vi "prep_outgoing_lineitem.vi"(2 "response":T1, 5 "error in (no error)":errorcluster) -> (15 "to_java":string, 17 "to_terminal":string, 19 "error out":errorcluster)   [LabVIEW 2016]
uses:
  controls/response.ctl
  controls/response_type.ctl
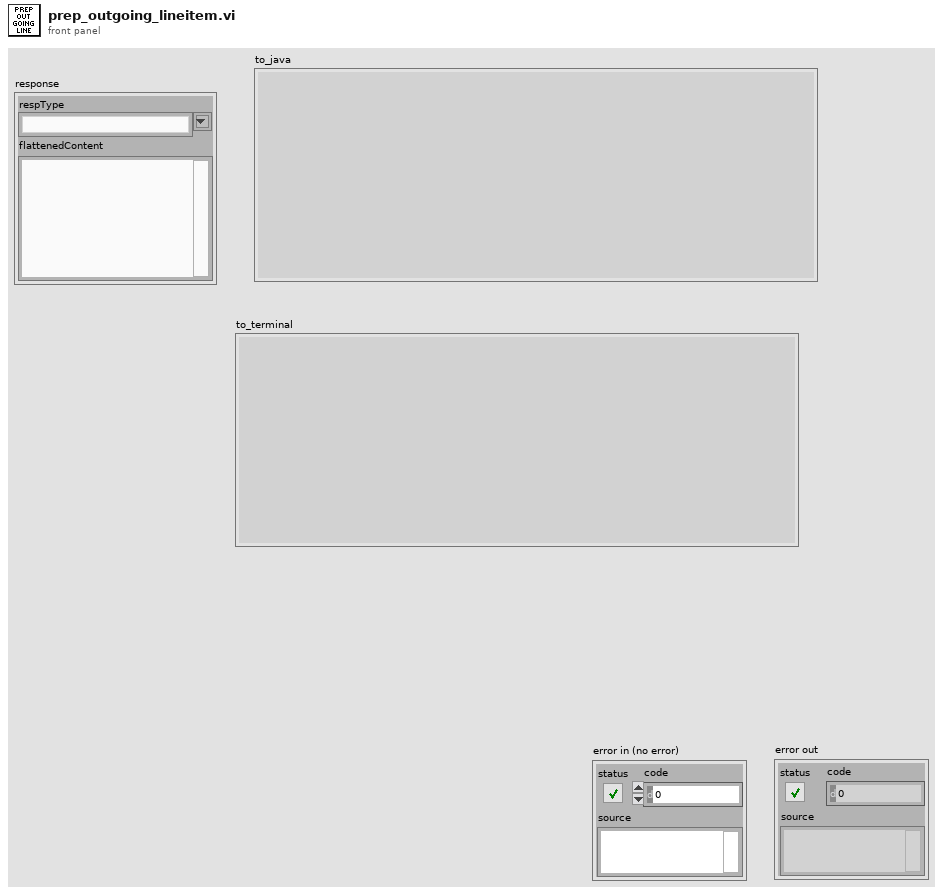
[diagram p1: front panel]
types:
  T1 = typedef "response.ctl" = cluster{"respType":T2, "flattenedContent":string}
  T2 = typedef "response_type.ctl" = string
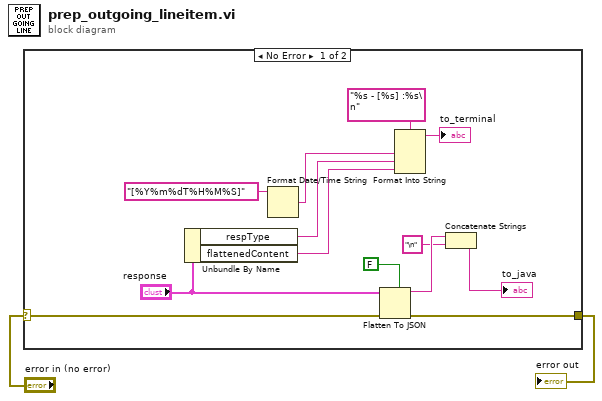
[diagram p0: block diagram]
diagram:
  n1 = case shown="No Error" "error in (no error)" {
    selector: "error in (no error)" -> [w8 w16]
    tunnel: [w7 w16] -> w1
    frame No Error {
      n2 = Unbundle By Name("response") -> ("respType"=w11:T2, "flattenedContent"=w12:string)
      n3 = Format Date/Time String(time format string (%c)="[%Y%m%dT%H%M%S]") -> (date/time string=w13:string)  [unwired: 2 in]
      n4 = Flatten To JSON(enable LabVIEW extensions? (T)=FALSE, anything="response", error in (no error)=w8) -> (JSON string=w5:string, 11:w7:errorcluster)
      n5 = Format Into String(format string="%s - [%s] :%s\n" ("time format string (%c)"), w13, w11, w12) -> (resulting string=→"to_terminal":string)  [unwired: 2 in, 1 out]
      n6 = Concatenate Strings(w5, "\n") -> (→"to_java":string)
    }
    frame Error {
    }
  }
  "error out" <- w1
